vi "load_image.vi"() -> ()   [LabVIEW 2021]
uses:
  <vilib>/picture/picture.llb/imagedata.ctl
panel:
  out "output":picture
  out "image data":T1
  out "Image":T2(plugin-control)
  out "File Data Type out":i32
  out "File Type out":string
  in  "input image":path
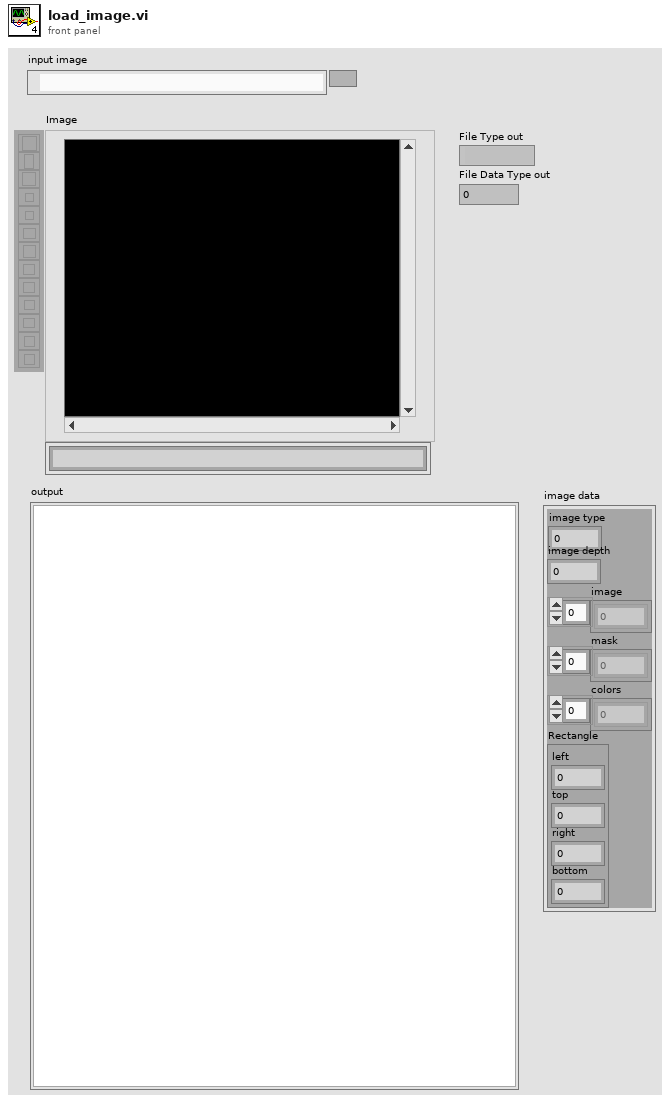
[diagram p1: front panel]
types:
  T1 = typedef "imagedata.ctl" = cluster{"image type":i32, "image depth":i32, "image":u8[], "mask":u8[], "colors":u32[], "Rectangle":cluster{"left":i16, "top":i16, "right":i16, "bottom":i16}}
  T2 = typedef "IMAQ Image.ctl" = refnum<image>
  T3 = typedef "Image Type" = u32
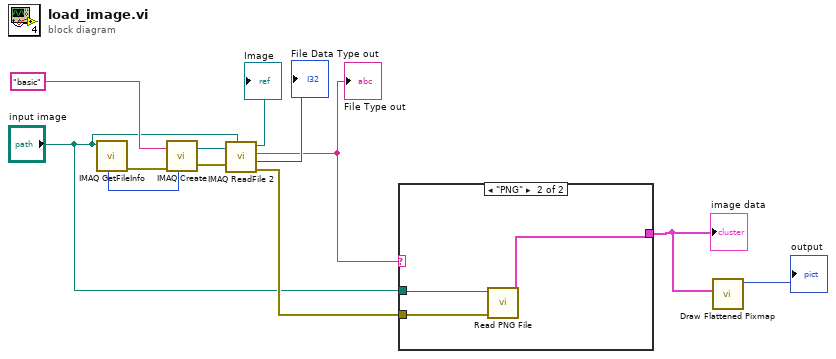
[diagram p0: block diagram]
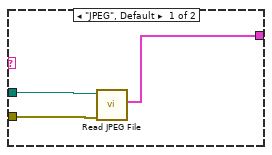
[diagram p2: hidden frame]
diagram:
  n1 = call "IMAQ GetFileInfo"("File Path"="input image") -> ("error out"=w10:errorcluster, "Image Type"=w12:T3)  [unwired: 4 in, 5 out]
  n2 = call "IMAQ Create"("Image Name"="basic", "Image Type"=w12, "error in (no error)"=w10) -> ("New Image"=w9:T2, "error out"=w8:errorcluster)  [unwired: 2 in]
  n3 = call "IMAQ ReadFile 2"("File Path"="input image", "error in (no error)"=w8, "Image"=w9) -> ("error out"=w4:errorcluster, "File Data Type out"=→"File Data Type out":i32, "File Type out"=w5:string, "Image Out"=→"Image":T2)  [unwired: 4 in, 1 out]
  "File Type out" <- w5
  n4 = case shown="\"PNG\"" w5 {
    tunnel: w4 -> [w14 w17]
    tunnel: "input image" -> [w15 w18]
    tunnel: [w13 w16] -> w2
    frame "JPEG", Default {
      n5 = call <vilib>:"Read JPEG File.vi"("error in (no error)"=w14, "path to JPEG file"=w15) -> ("image data"=w13:T1)  [unwired: 7 in, 2 out]
    }
    frame "PNG" {
      n6 = call <vilib>:"Read PNG File.vi"("error in (no error)"=w17, "path to PNG file"=w18) -> ("image data"=w16:T1)  [unwired: 7 in, 2 out]
    }
  }
  "image data" <- w2
  n7 = call <vilib>:"Draw Flattened Pixmap.vi"("image data"=w2) -> ("new picture"=→"output":picture)  [unwired: 8 in]
